vi "Read Config Digitals.vi"(0 "connection ID":refnum<k16>, 1 "address":u32, 2 "port":u16, 9 "timeout ms (1000)":i32=1000, 11 "error in (no error)":errorcluster) -> (4 "connection ID out":refnum<k16>, 6 "received data":string, 8 "Digital Mode":T1[](array[typedef]) items=["Output"=79, "Input_Pullup"=80, "Input"=73], 15 "error out":errorcluster)   [LabVIEW 2016, in "instr.lvlib"]
doc: "Reads all digital modes and returns them as array. Batch operation."
uses:
  instr.lvlib
  Digital Mode.ctl
panel:
  out "Send String":string
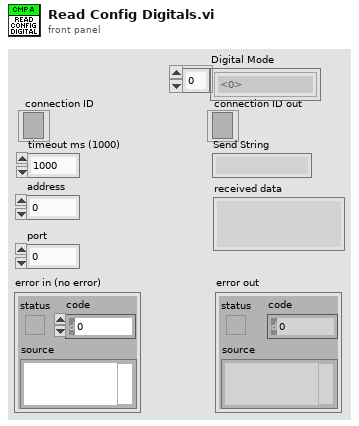
[diagram p1: front panel]
types:
  T1 = typedef "instr.lvlib/Digital Mode.ctl" = u16
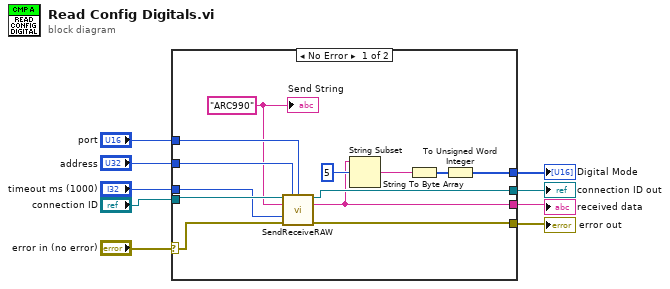
[diagram p0: block diagram]
diagram:
  n1 = case shown="No Error" "error in (no error)" {
    selector: "error in (no error)" -> [w10 w24]
    tunnel: [w22 w24] -> w9
    tunnel: "timeout ms (1000)" -> [w19 _]
    tunnel: "connection ID" -> [w20 w23]
    tunnel: [w21 w23] -> w5
    tunnel: "address" -> [w18 _]
    tunnel: "port" -> [w17 _]
    tunnel: [w14 _] -> w2
    tunnel: [w11 _] -> w1
    frame No Error {
      w16 = "ARC990" ("data in")
      n2 = call "SendReceiveRAW.vi"("connection ID"=w20, "address"=w18, "port"=w17, "RAW data in"=w16, "timeout ms (1000)"=w19, "error in (no error)"=w10) -> ("connection ID out"=w21:refnum<k16>, "received data"=w14:string, "error out"=w22:errorcluster)  [unwired: 7 in]
      n3 = String Subset(string=w14, offset (0)=5 ("offset")) -> (substring=w13:string)  [unwired: 1 in]
      n4 = String To Byte Array(string=w13) -> (unsigned byte array=w12:u8[])
      n5 = To Unsigned Word Integer(number=w12) -> (unsigned 16bit integer=w11:u16[])
      "Send String" <- w16
    }
    frame Error {
    }
  }
  "error out" <- w9
  "received data" <- w2
  "connection ID out" <- w5
  "Digital Mode" <- w1
